vi "CCE T027 SubVI01.vi"(10 "CAPA DE COLOR":T1(ring), 11 "RUTA DE IMAGEN":path) -> (3 "Array":u8[][](array[numeric]))   [LabVIEW 2020]
doc: "Ceballos Conde Emanuel 4MV6 Sistemas de visión artificial 2022/1\neste vi permite hacer la conversion obtener una capa de las componentes RGB, HSV,CMY o escala de grisis,"
panel:
  # "Ceballos Conde Emanuel\n4MV6\nSistemas de visión artificial\n2022/1"
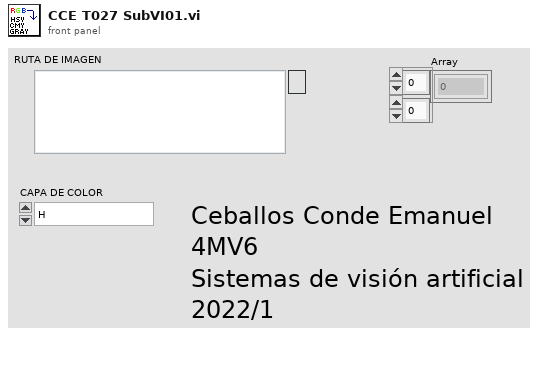
[diagram p1: front panel]
types:
  T1 = enum16{"H", "S", "V", "C", "M", "Y", "R", "G", "B", "RGB2GRAY MATLAB"}
  T2 = typedef "IMAQ Image.ctl" = refnum<image>
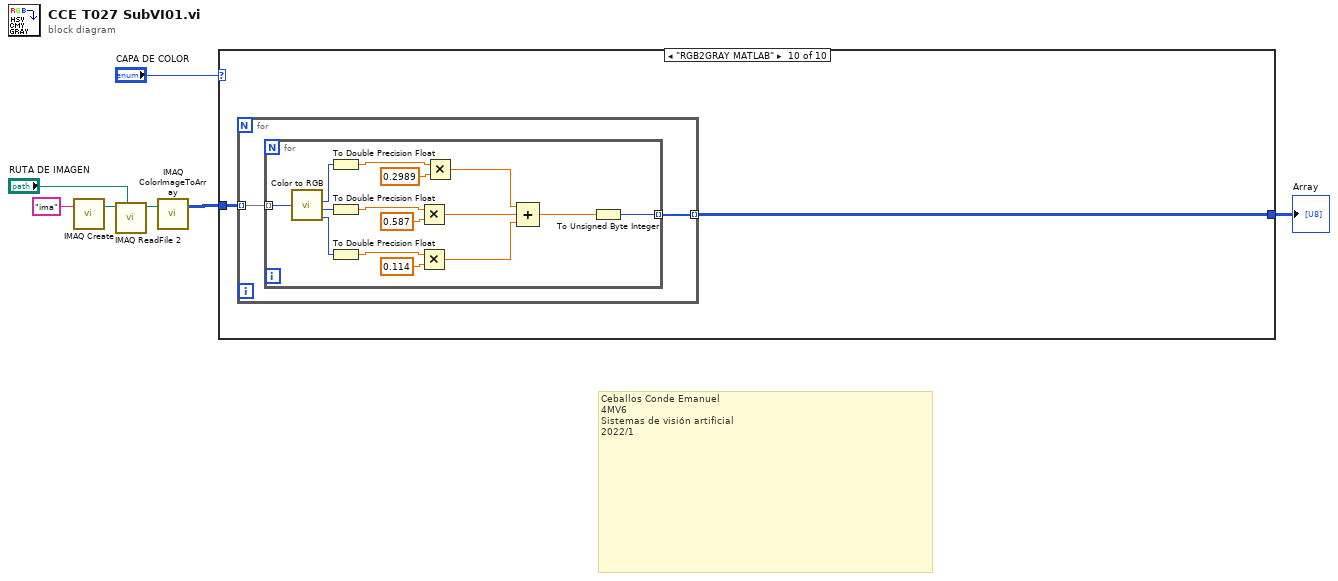
[diagram p0: block diagram]
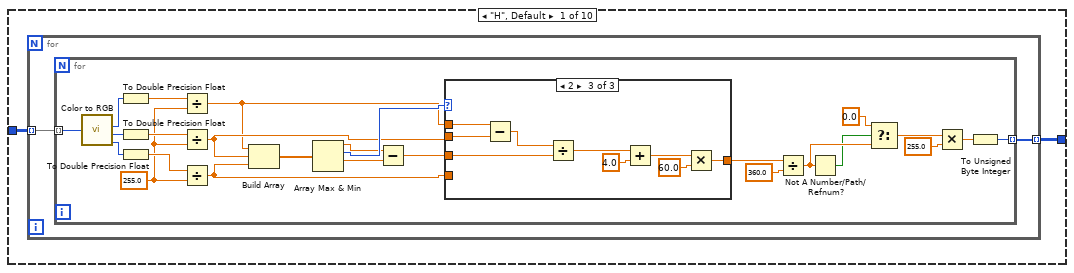
[diagram p2: hidden frame]
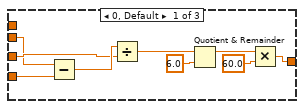
[diagram p3: hidden frame]
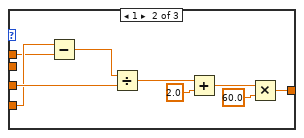
[diagram p4: hidden frame]
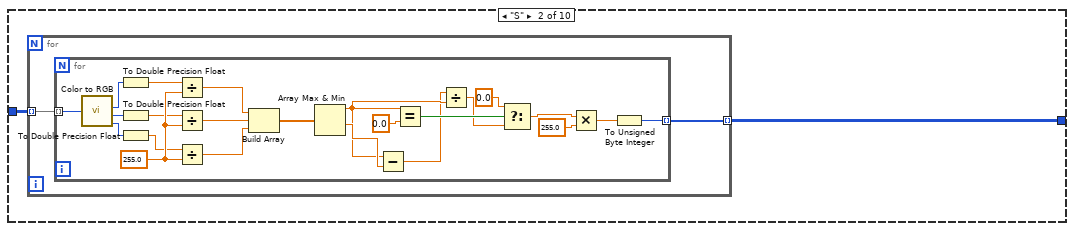
[diagram p5: hidden frame]
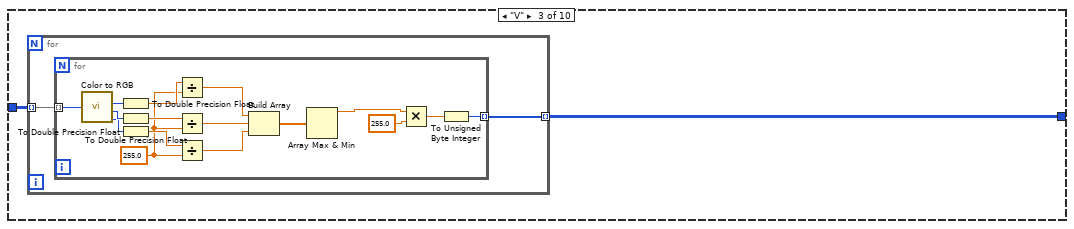
[diagram p6: hidden frame]
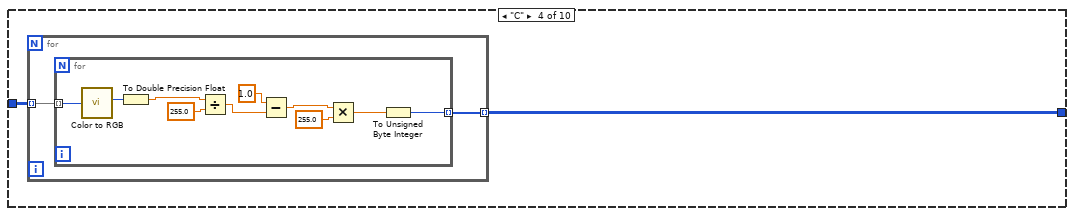
[diagram p7: hidden frame]
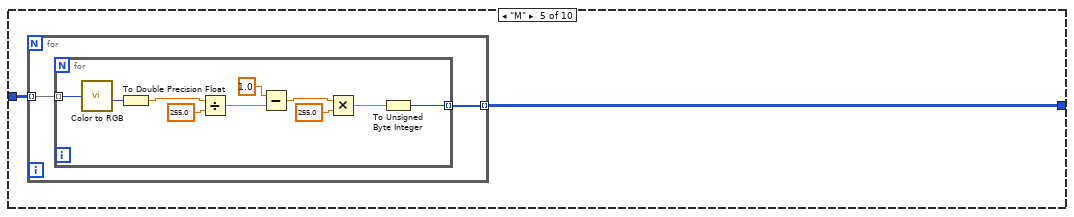
[diagram p8: hidden frame]
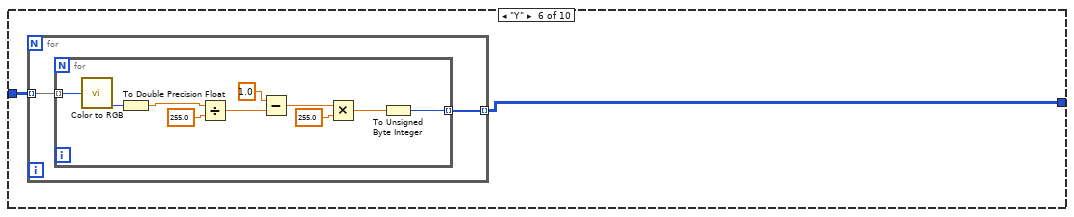
[diagram p9: hidden frame]
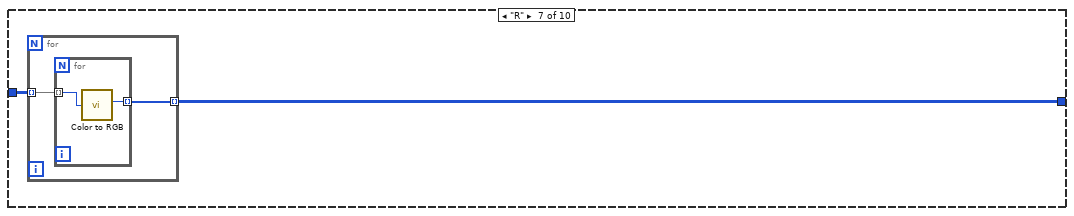
[diagram p10: hidden frame]
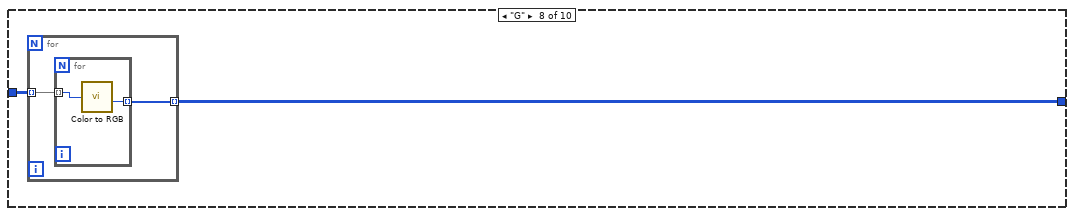
[diagram p11: hidden frame]
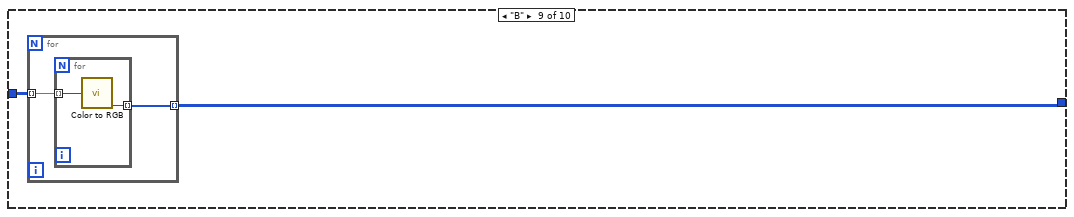
[diagram p12: hidden frame]
diagram:
  # "Ceballos Conde Emanuel\n4MV6\nSistemas de visión artificial\n2022/1"
  n1 = call "IMAQ Create"("Image Name"="ima") -> ("New Image"=w5:T2)  [unwired: 4 in, 1 out]
  n2 = call "IMAQ ReadFile 2"("File Path"="RUTA DE IMAGEN", "Image"=w5) -> ("Image Out"=w3:T2)  [unwired: 5 in, 4 out]
  n3 = call "IMAQ ColorImageToArray"("Image"=w3) -> ("Image Pixels (U32)"=w2:u32[][])  [unwired: 3 in, 2 out]
  n4 = case shown="\"RGB2GRAY MATLAB\"" "CAPA DE COLOR" {
    tunnel: [w9 w65 w92 w111 w125 w139 w153 w159 w165 w171] -> w1
    tunnel: w2 -> [w8 w64 w91 w112 w126 w140 w154 w160 w166 w172]
    frame "H", Default {
      n5 = for {
        tunnel: [w11] -> w9 mode=indexing
        tunnel: w8 -> [w10] mode=indexing
        n6 = for {
          tunnel: [w12] -> w11 mode=indexing
          tunnel: w10 -> [w19] mode=indexing
          w22 = 255.0 ("y")
          n7 = call <vilib>:"Color to RGB.vi"("Color"=w19) -> ("R"=w18:u8, "G"=w17:u8, "B"=w16:u8)  [unwired: 1 out]
          n8 = To Double Precision Float(number=w18) -> (double precision float=w23:dbl)
          n9 = To Double Precision Float(number=w17) -> (double precision float=w24:dbl)
          n10 = To Double Precision Float(number=w16) -> (double precision float=w25:dbl)
          n11 = Divide(x=w23, y=w22) -> (x/y=w31:dbl)
          n12 = Divide(x=w24, y=w22) -> (x/y=w32:dbl)
          n13 = Divide(x=w25, y=w22) -> (x/y=w33:dbl)
          n14 = Build Array(w31, w32, w33) -> (w26:dbl[])
          n15 = Array Max & Min(array=w26) -> (max value=w28:dbl, max index (indices)=w36:i32, min value=w27:dbl)  [unwired: 1 out]
          n16 = Subtract(x=w28, y=w27) -> (x-y=w29:dbl)
          n17 = case shown="2" w36 {
            tunnel: [w39 w48 w57] -> w30
            tunnel: w32 -> [w38 _ w55]
            tunnel: w33 -> [w37 w47 _]
            tunnel: w29 -> [w44 w53 w62]
            tunnel: w31 -> [_ w46 w56]
            frame 0, Default {
              n18 = Subtract(x=w38, y=w37) -> (x-y=w45:dbl)
              n19 = Divide(x=w45, y=w44) -> (x/y=w43:dbl)
              n20 = Quotient & Remainder(x=w43, y=6.0) -> (x-y*floor(x/y)=w40:dbl)  [unwired: 1 out]
              n21 = Multiply(x=w40, y=60.0) -> (x*y=w39:dbl)
            }
            frame 1 {
              n22 = Subtract(x=w47, y=w46) -> (x-y=w54:dbl)
              n23 = Divide(x=w54, y=w53) -> (x/y=w52:dbl)
              n24 = Add(x=w52, y=2.0) -> (x+y=w49:dbl)
              n25 = Multiply(x=w49, y=60.0) -> (x*y=w48:dbl)
            }
            frame 2 {
              n26 = Subtract(x=w56, y=w55) -> (x-y=w63:dbl)
              n27 = Divide(x=w63, y=w62) -> (x/y=w61:dbl)
              n28 = Add(x=w61, y=4.0) -> (x+y=w58:dbl)
              n29 = Multiply(x=w58, y=60.0) -> (x*y=w57:dbl)
            }
          }
          n30 = Divide(x=w30, y=360.0) -> (x/y=w35:dbl)
          n31 = Not A Number/Path/Refnum?(number/path/refnum=w35) -> (NaN/Path/Refnum?=w34:bool)
          n32 = Select(t=0.0, s=w34, f=w35) -> (s? t:f=w14:dbl)
          n33 = Multiply(x=w14, y=255.0) -> (x*y=w15:dbl)
          n34 = To Unsigned Byte Integer(number=w15) -> (unsigned 8bit integer=w12:u8)
        }
      }
    }
    frame "S" {
      n35 = for {
        tunnel: [w67] -> w65 mode=indexing
        tunnel: w64 -> [w66] mode=indexing
        n36 = for {
          tunnel: [w68] -> w67 mode=indexing
          tunnel: w66 -> [w75] mode=indexing
          w90 = 255.0 ("y")
          n37 = call <vilib>:"Color to RGB.vi"("Color"=w75) -> ("R"=w74:u8, "G"=w73:u8, "B"=w72:u8)  [unwired: 1 out]
          n38 = To Double Precision Float(number=w74) -> (double precision float=w89:dbl)
          n39 = To Double Precision Float(number=w73) -> (double precision float=w88:dbl)
          n40 = To Double Precision Float(number=w72) -> (double precision float=w87:dbl)
          n41 = Divide(x=w89, y=w90) -> (x/y=w78:dbl)
          n42 = Divide(x=w88, y=w90) -> (x/y=w77:dbl)
          n43 = Divide(x=w87, y=w90) -> (x/y=w76:dbl)
          n44 = Build Array(w78, w77, w76) -> (w86:dbl[])
          n45 = Array Max & Min(array=w86) -> (max value=w80:dbl, min value=w82:dbl)  [unwired: 2 out]
          n46 = Subtract(x=w80, y=w82) -> (x-y=w79:dbl)
          n47 = Equal?(x=w80, y=0.0) -> (x = y?=w84:bool)
          n48 = Divide(x=w79, y=w80) -> (x/y=w81:dbl)
          n49 = Select(t=0.0, s=w84, f=w81) -> (s? t:f=w70:dbl)
          n50 = Multiply(x=w70, y=255.0) -> (x*y=w69:dbl)
          n51 = To Unsigned Byte Integer(number=w69) -> (unsigned 8bit integer=w68:u8)
        }
      }
    }
    frame "V" {
      n52 = for {
        tunnel: [w94] -> w92 mode=indexing
        tunnel: w91 -> [w93] mode=indexing
        n53 = for {
          tunnel: [w95] -> w94 mode=indexing
          tunnel: w93 -> [w102] mode=indexing
          w104 = 255.0 ("y")
          n54 = call <vilib>:"Color to RGB.vi"("Color"=w102) -> ("R"=w101:u8, "G"=w100:u8, "B"=w99:u8)  [unwired: 1 out]
          n55 = To Double Precision Float(number=w101) -> (double precision float=w105:dbl)
          n56 = To Double Precision Float(number=w100) -> (double precision float=w106:dbl)
          n57 = To Double Precision Float(number=w99) -> (double precision float=w107:dbl)
          n58 = Divide(x=w105, y=w104) -> (x/y=w109:dbl)
          n59 = Divide(x=w106, y=w104) -> (x/y=w103:dbl)
          n60 = Divide(x=w107, y=w104) -> (x/y=w110:dbl)
          n61 = Build Array(w109, w103, w110) -> (w108:dbl[])
          n62 = Array Max & Min(array=w108) -> (max value=w97:dbl)  [unwired: 3 out]
          n63 = Multiply(x=w97, y=255.0) -> (x*y=w96:dbl)
          n64 = To Unsigned Byte Integer(number=w96) -> (unsigned 8bit integer=w95:u8)
        }
      }
    }
    frame "C" {
      n65 = for {
        tunnel: w112 -> [w114] mode=indexing
        tunnel: [w113] -> w111 mode=indexing
        n66 = for {
          tunnel: w114 -> [w124] mode=indexing
          tunnel: [w115] -> w113 mode=indexing
          n67 = call <vilib>:"Color to RGB.vi"("Color"=w124) -> ("R"=w123:u8)  [unwired: 3 out]
          n68 = To Double Precision Float(number=w123) -> (double precision float=w119:dbl)
          n69 = Divide(x=w119, y=255.0) -> (x/y=w121:dbl)
          n70 = Subtract(x=1.0, y=w121) -> (x-y=w118:dbl)
          n71 = Multiply(x=w118, y=255.0) -> (x*y=w116:dbl)
          n72 = To Unsigned Byte Integer(number=w116) -> (unsigned 8bit integer=w115:u8)
        }
      }
    }
    frame "M" {
      n73 = for {
        tunnel: w126 -> [w128] mode=indexing
        tunnel: [w127] -> w125 mode=indexing
        n74 = for {
          tunnel: w128 -> [w138] mode=indexing
          tunnel: [w130] -> w127 mode=indexing
          n75 = call <vilib>:"Color to RGB.vi"("Color"=w138) -> ("G"=w129:u8)  [unwired: 3 out]
          n76 = To Double Precision Float(number=w129) -> (double precision float=w134:dbl)
          n77 = Divide(x=w134, y=255.0) -> (x/y=w136:dbl)
          n78 = Subtract(x=1.0, y=w136) -> (x-y=w133:dbl)
          n79 = Multiply(x=w133, y=255.0) -> (x*y=w131:dbl)
          n80 = To Unsigned Byte Integer(number=w131) -> (unsigned 8bit integer=w130:u8)
        }
      }
    }
    frame "Y" {
      n81 = for {
        tunnel: w140 -> [w142] mode=indexing
        tunnel: [w141] -> w139 mode=indexing
        n82 = for {
          tunnel: w142 -> [w152] mode=indexing
          tunnel: [w144] -> w141 mode=indexing
          n83 = call <vilib>:"Color to RGB.vi"("Color"=w152) -> ("B"=w143:u8)  [unwired: 3 out]
          n84 = To Double Precision Float(number=w143) -> (double precision float=w148:dbl)
          n85 = Divide(x=w148, y=255.0) -> (x/y=w150:dbl)
          n86 = Subtract(x=1.0, y=w150) -> (x-y=w147:dbl)
          n87 = Multiply(x=w147, y=255.0) -> (x*y=w145:dbl)
          n88 = To Unsigned Byte Integer(number=w145) -> (unsigned 8bit integer=w144:u8)
        }
      }
    }
    frame "R" {
      n89 = for {
        tunnel: w154 -> [w156] mode=indexing
        tunnel: [w155] -> w153 mode=indexing
        n90 = for {
          tunnel: w156 -> [w158] mode=indexing
          tunnel: [w157] -> w155 mode=indexing
          n91 = call <vilib>:"Color to RGB.vi"("Color"=w158) -> ("R"=w157:u8)  [unwired: 3 out]
        }
      }
    }
    frame "G" {
      n92 = for {
        tunnel: w160 -> [w162] mode=indexing
        tunnel: [w161] -> w159 mode=indexing
        n93 = for {
          tunnel: w162 -> [w164] mode=indexing
          tunnel: [w163] -> w161 mode=indexing
          n94 = call <vilib>:"Color to RGB.vi"("Color"=w164) -> ("G"=w163:u8)  [unwired: 3 out]
        }
      }
    }
    frame "B" {
      n95 = for {
        tunnel: w166 -> [w168] mode=indexing
        tunnel: [w167] -> w165 mode=indexing
        n96 = for {
          tunnel: w168 -> [w170] mode=indexing
          tunnel: [w169] -> w167 mode=indexing
          n97 = call <vilib>:"Color to RGB.vi"("Color"=w170) -> ("B"=w169:u8)  [unwired: 3 out]
        }
      }
    }
    frame "RGB2GRAY MATLAB" {
      n98 = for {
        tunnel: w172 -> [w174] mode=indexing
        tunnel: [w173] -> w171 mode=indexing
        n99 = for {
          tunnel: w174 -> [w189] mode=indexing
          tunnel: [w178] -> w173 mode=indexing
          n100 = call <vilib>:"Color to RGB.vi"("Color"=w189) -> ("R"=w188:u8, "G"=w187:u8, "B"=w186:u8)  [unwired: 1 out]
          n101 = To Double Precision Float(number=w188) -> (double precision float=w177:dbl)
          n102 = To Double Precision Float(number=w187) -> (double precision float=w176:dbl)
          n103 = To Double Precision Float(number=w186) -> (double precision float=w175:dbl)
          n104 = Multiply(x=w176, y=0.587) -> (x*y=w181:dbl)
          n105 = Multiply(x=w175, y=0.114) -> (x*y=w180:dbl)
          n106 = Multiply(x=w177, y=0.2989) -> (x*y=w182:dbl)
          n107 = Compound Arithmetic op=ADD(w182, w181, w180) -> (w179:dbl)
          n108 = To Unsigned Byte Integer(number=w179) -> (unsigned 8bit integer=w178:u8)
        }
      }
    }
  }
  "Array" <- w1
